vi "EndTest.vi"(7 "Time":dbl, 8 "error in (no error)":errorcluster, 10 "Test":refnum<class "Test.lvclass">, 11 "ResultTreeListener in":refnum<class "ResultTreeListener.lvclass">) -> (0 "error out":errorcluster, 3 "ResultTreeListener out":refnum<class "ResultTreeListener.lvclass">)   [LabVIEW 2019, in "ResultTreeListener.lvclass"]
doc: "A test ended."
uses:
  ResultTreeListener.lvclass
  ResultTreeListener.lvclass/ResultTreeListener.ctl
  ResultTree/ResultTree.lvclass
  Test/Test.lvclass
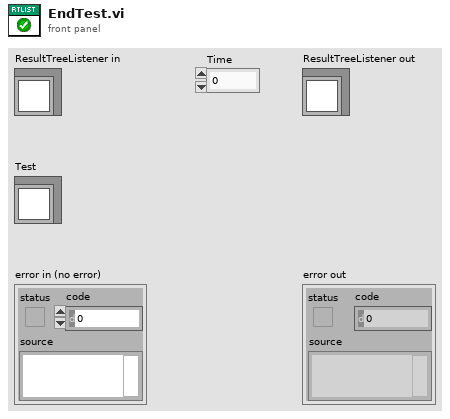
[diagram p1: front panel]
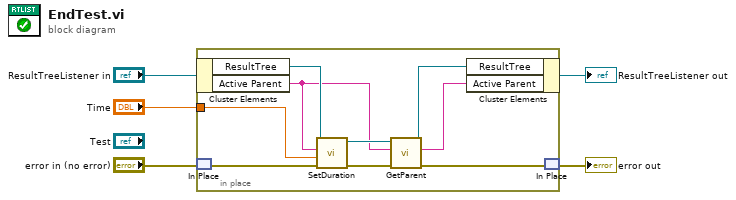
[diagram p0: block diagram]
diagram:
  n1 = in-place {
    in-place-border: "Time" -> [w6]
    n2 = in-place-cluster #1("ResultTreeListener in") -> ("ResultTree"=w9:refnum<class "ResultTree.lvclass">, "Active Parent"=w7:string)
    n3 = in-place-match #2("error in (no error)") -> (w13:errorcluster)
    n4 = call "SetDuration.vi"("error in (no error)"=w13, "Duration [s]"=w6, "Tag Name"=w7, "ResultTree in"=w9) -> ("error out"=w10:errorcluster, "ResultTree out"=w8:refnum<class "ResultTree.lvclass">)  [unwired: 6 in]
    n5 = call "GetParent.vi"("error in (no error)"=w10, "Tag"=w7, "ResultTree in"=w8) -> ("error out"=w12:errorcluster, "Parent Tag"=w11:string, "ResultTree out"=w14:refnum<class "ResultTree.lvclass">)  [unwired: 6 in]
    n6 = in-place-cluster #1("ResultTree"=w14, "Active Parent"=w11) -> (→"ResultTreeListener out":refnum<class "ResultTreeListener.lvclass">)
    n7 = in-place-match #2(w12) -> (→"error out":errorcluster)
  }
